vi "Wait for OPC.vi"(8 "error in (no error)":errorcluster, 10 "Time Target (s)":dbl=65.0 format="%#_13g", 11 "SpecA_ESA.lvclass.In":refnum<class "SpecA_ESA.lvclass">) -> (0 "error out":errorcluster, 2 "OPC?":bool, 3 "SpecA_ESA.lvclass.Out":refnum<class "SpecA_ESA.lvclass">)   [LabVIEW 2014, in "SpecA_ESA.lvclass"]
doc: "Waits for the current operation to finish. This VI should be called after Initiate VI.\n\n<B>Note:</B> \n\nUse this VI only with other low-level VIs. The high-level VIs automatically incorporate this functionality. This VI does not check the instrument status."
uses:
  SpecA_ESA.lvclass
  SpecA_ESA.lvclass/SpecA_ESA.ctl
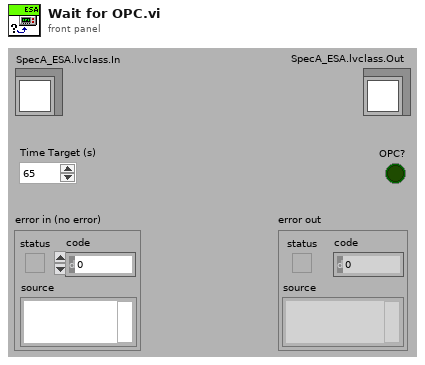
[diagram p1: front panel]
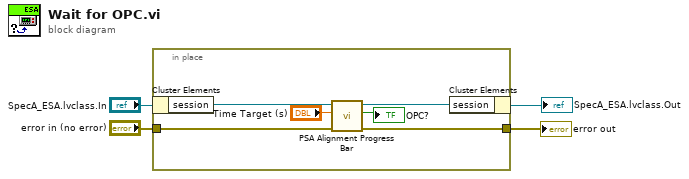
[diagram p0: block diagram]
diagram:
  n1 = in-place {
    in-place-border: "error in (no error)" -> [w10]
    in-place-border: [w9] -> w1
    n2 = in-place-cluster #1("SpecA_ESA.lvclass.In") -> ("session"=w8:refnum<visa-resource-name>)
    n3 = call "PSA Alignment Progress Bar.vi"("error in (no error)"=w10, "Time Target (s)"="Time Target (s)", "VISA resource in"=w8) -> ("error out"=w9:errorcluster, "Complete?"=→"OPC?":bool, "VISA resource out"=w6:refnum<visa-resource-name>)  [unwired: 6 in]
    n4 = in-place-cluster #1("session"=w6) -> (→"SpecA_ESA.lvclass.Out":refnum<class "SpecA_ESA.lvclass">)
  }
  "error out" <- w1
